vi "setFrontPanelCommand.vi"(8 "error in (no error)":errorcluster, 11 "TEI9150 in":refnum<class "TEI9150.lvclass">) -> (0 "error out":errorcluster, 3 "TEI9150 out":refnum<class "TEI9150.lvclass">)   [LabVIEW 2015, in "TEI9150.lvclass"]
uses:
  TEI9150.lvclass
  TEI9150.lvclass/TEI9150.ctl
  <userlib>/Common/SerialProtocols/SerialCommunicator/SerialCommunicator.lvclass
panel:
  out "Front Panel Set Command":string
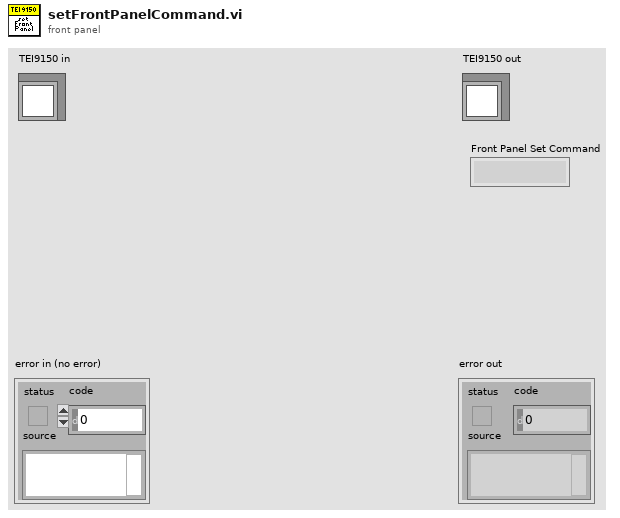
[diagram p1: front panel]
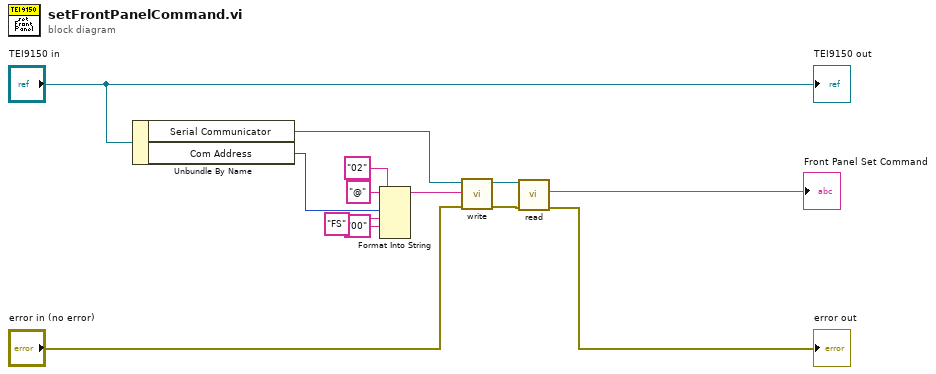
[diagram p0: block diagram]
diagram:
  n1 = Unbundle By Name("TEI9150 in") -> ("Serial Communicator"=w12:refnum<class "SerialCommunicator.lvclass">, "Com Address"=w10:u8)
  n2 = Format Into String(initial string="@", w10, "FS" ("input 2"), "00" ("input 3"), "02" ("input 4")) -> (resulting string=w8:string)  [unwired: 2 in, 1 out]
  n3 = call-dynamic "write.vi"("error in (no error)"="error in (no error)", "writeString"=w8, "SerialCommunicator in"=w12) -> ("error out"=w7:errorcluster, "SerialCommunicator out"=w6:refnum<class "SerialCommunicator.lvclass">)  [unwired: 7 in]
  n4 = call-dynamic "read.vi"("error in (no error)"=w7, "SerialCommunicator in"=w6) -> ("error out"=→"error out":errorcluster, "stringRead"=→"Front Panel Set Command":string)  [unwired: 7 in, 1 out]
  "TEI9150 out" <- "TEI9150 in"
